vi "Write Post AOV Values.vi"(8 "error in":errorcluster, 11 "DAC HeatFlow AOV in":refnum<class "DAC HeatFlow AOV.lvclass">) -> (0 "error out":errorcluster, 3 "DAC HeatFlow AOV out":refnum<class "DAC HeatFlow AOV.lvclass">)   [LabVIEW 2019, in "DAC.lvlib" / "DAC HeatFlow AOV.lvclass"]
uses:
  DAC HeatFlow AOV.lvclass
  Results/Results Method.ctl
  Results/Results.lvlib
  Results/Heat Flow Results/Heat Flow Results.lvclass
  <vilib>/DAQmx/write.llb/DAQmx Write (Analog 1D DBL NChan 1Samp).vi
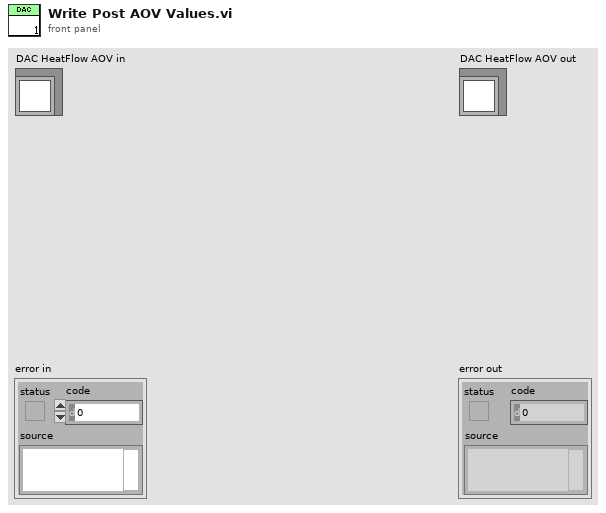
[diagram p1: front panel]
types:
  T1 = typedef "Results.lvlib/Results Method.ctl" = enum16{"Get", "Set"}
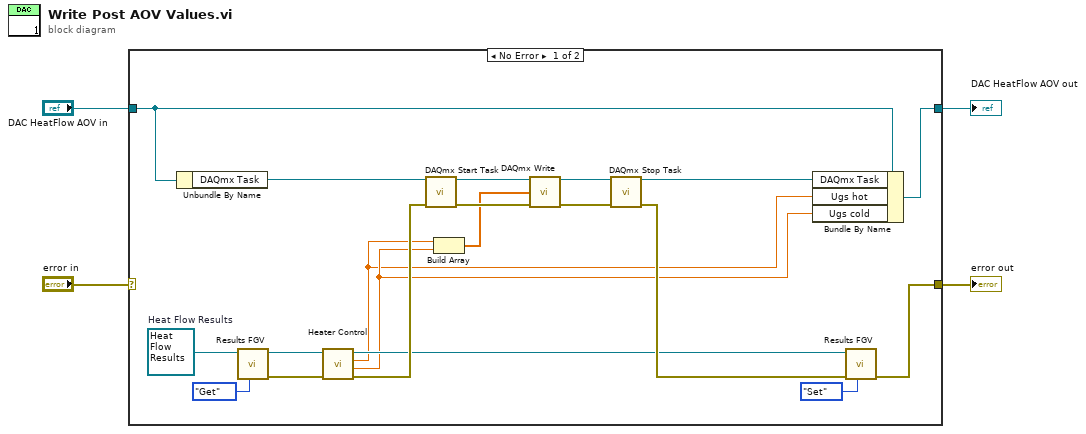
[diagram p0: block diagram]
diagram:
  n1 = case shown="No Error" "error in" {
    selector: "error in" -> [_ w26]
    tunnel: [w13 w26] -> w3
    tunnel: [w24 w25] -> w1
    tunnel: "DAC HeatFlow AOV in" -> [w23 w25]
    frame No Error {
      w15 = refnum<class "Heat Flow Results.lvclass"> refnum  # Heat Flow Results
      n2 = Unbundle By Name(w23) -> ("DAQmx Task"=w22:refnum<k21>)
      n3 = call-dynamic "Results FGV.vi"("Method"=Results_Method."Get", "Results in"=w15) -> ("error out"=w11:errorcluster, "Results out"=w10:refnum<class "Heat Flow Results.lvclass">)  [unwired: 8 in]
      n4 = call "Heater Control.vi"("error in"=w11, "HeatFlow Results in"=w10) -> ("error out"=w9:errorcluster, "Ugs Cold"=w6:dbl, "Ugs Hot"=w5:dbl, "HeatFlow Results out"=w8:refnum<class "Heat Flow Results.lvclass">)  [unwired: 6 in]
      n5 = call <vilib>:"DAQmx Start Task.vi"("task/channels in"=w22, "error in"=w9) -> ("task out"=w21:refnum<k21>, "error out"=w19:errorcluster)  [unwired: 12 in]
      n6 = Build Array(w5, w6) -> (w7:dbl[])
      n7 = call-poly <vilib>:"DAQmx Write.vi"("task/channels in"=w21, "data"=w7, "error in"=w19) -> ("task out"=w20:refnum<k21>, "error out"=w18:errorcluster)  [unwired: 10 in, 1 out]
      n8 = call <vilib>:"DAQmx Stop Task.vi"("task/channels in"=w20, "error in"=w18) -> ("task out"=w12:refnum<k21>, "error out"=w14:errorcluster)  [unwired: 12 in]
      n9 = Bundle By Name(cluster=w23, "DAQmx Task"=w12, "Ugs hot"=w5, "Ugs cold"=w6) -> (w24:refnum<class "DAC HeatFlow AOV.lvclass">)
      n10 = call-dynamic "Results FGV.vi"("Method"=Results_Method."Set", "error in"=w14, "Results in"=w8) -> ("error out"=w13:errorcluster)  [unwired: 7 in, 1 out]
    }
    frame Error {
    }
  }
  "error out" <- w3
  "DAC HeatFlow AOV out" <- w1
